vi "Initialize.vi"(8 "error in (no error)":errorcluster, 10 "Laser Configuration":T1, 11 "Coherent Laser in":refnum<class "Coherent Laser.lvclass">) -> (0 "error out":errorcluster, 3 "Coherent Laser out":refnum<class "Coherent Laser.lvclass">)   [LabVIEW 2023, in "Coherent Laser.lvlib" / "Coherent Laser.lvclass"]
uses:
  Coherent Laser.lvclass
  Resources/Type Defs/Laser Configuration.ctl
  Coherent Laser.lvclass/Coherent Laser.ctl
  Resources/GLOBAL/GLOBAL Debug.vi
  <vilib>/Utility/error.llb/Error Cluster From Error Code.vi
  <vilib>/ErrorRing/Error Ring.xnode
  <vilib>/Instr/_visa.llb/VISA Configure Serial Port (Instr).vi
  Coherent Laser.lvlib
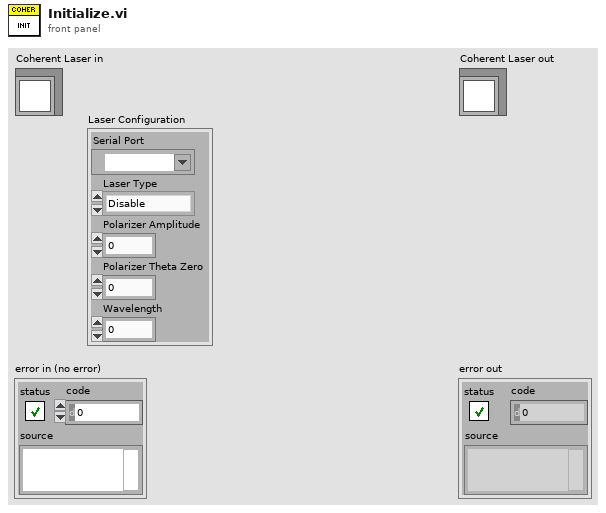
[diagram p1: front panel]
types:
  T1 = typedef "Laser Configuration.ctl" = cluster{"Serial Port":refnum<visa-resource-name>, "Laser Type":enum16{"Disable", "Laser Quantum", "Coherent OBIS", "PRM1-Z8", "Coherent HOPS"}, "Polarizer Amplitude":dbl, "Polarizer Theta Zero":dbl, "Wavelength":u16}
  T2 = enum16{"Disable", "Laser Quantum", "Coherent OBIS", "PRM1-Z8", "Coherent HOPS"}
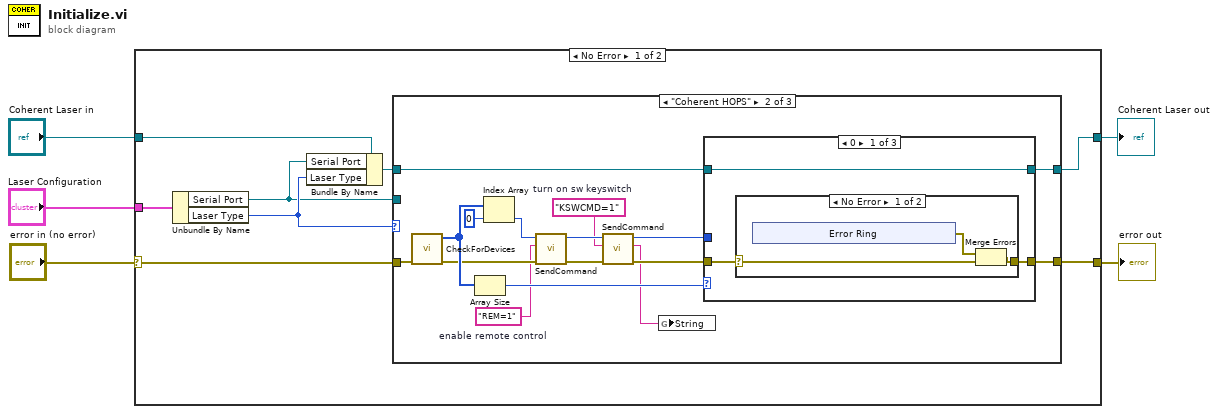
[diagram p0: block diagram]
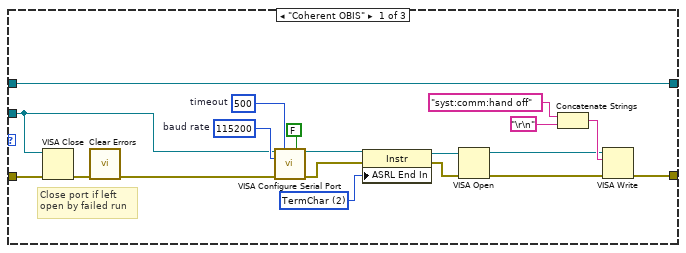
[diagram p2: hidden frame]
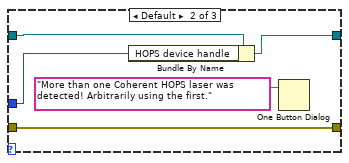
[diagram p4: hidden frame]
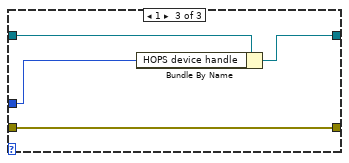
[diagram p5: hidden frame]
diagram:
  n1 = case shown="No Error" "error in (no error)" {
    selector: "error in (no error)" -> [w13 w72]
    tunnel: [w7 w72] -> w4
    tunnel: [w6 w71] -> w2
    tunnel: "Coherent Laser in" -> [w10 w71]
    tunnel: "Laser Configuration" -> [w12 _]
    frame No Error {
      n2 = Unbundle By Name(w12) -> ("Serial Port"=w8:refnum<visa-resource-name>, "Laser Type"=w9:T2)
      n3 = Bundle By Name(cluster=w10, "Serial Port"=w8, "Laser Type"=w9) -> (w11:refnum<class "Coherent Laser.lvclass">)
      n4 = case shown="\"Coherent HOPS\"" w9 {
        tunnel: w8 -> [w15 _ _]
        tunnel: w13 -> [w18 w48 w70]
        tunnel: [w27 w44 w70] -> w7
        tunnel: w11 -> [w14 w43 w69]
        tunnel: [w14 w42 w69] -> w6
        frame "Coherent OBIS" {
          w21 = u16 2 items=["None", "Last Bit", "TermChar"] ("Serial Settings:End Mode for Reads")
          w26 = u32 500  # timeout
          w28 = u32 115200  # baud rate
          # "Close port if left\nopen by failed run"
          n5 = VISA Close(VISA resource name=w15, error in (no error)=w18) -> (error out=w17:errorcluster)
          n6 = call <vilib>:"Clear Errors.vi"("error in (no error)"=w17) -> ("error out"=w16:errorcluster)  [unwired: 5 in, 1 out]
          n7 = call-poly "VISA Configure Serial Port"("VISA resource name"=w15, "timeout (10sec)"=w26, "Enable Termination\nChar (T)"=FALSE ("Enable Termination\nChar (T)"), "baud rate (9600)"=w28, "error in (no error)"=w16) -> ("VISA resource name out"=w25:refnum<visa-resource-name>, "error out"=w22:errorcluster)  [unwired: 9 in]
          n8 = property class="Instr"(reference=w25, error in=w22, "ASRL End In"=w21) -> (reference out=w24:refnum<visa-resource-name>, error out=w23:errorcluster)
          n9 = VISA Open(error in (no error)=w23, VISA resource name=w24) -> (VISA resource name=w19:refnum<visa-resource-name>, error out=w20:errorcluster)  [unwired: 3 in]
          n10 = Concatenate Strings("syst:comm:hand off" ("write to laser"), "\r\n") -> (w32:string)
          n11 = VISA Write(VISA resource name=w19, write buffer=w32, error in (no error)=w20) -> (error out=w27:errorcluster)  [unwired: 2 out]
        }
        frame "Coherent HOPS" {
          w33 = "KSWCMD=1"  # turn on sw keyswitch
          w39 = "REM=1"  # enable remote control
          n12 = call "CheckForDevices.vi"("error in"=w48) -> ("error out"=w41:errorcluster, "Device Handles"=w45:u64[])  [unwired: 6 in, 1 out]
          n13 = Array Size(array=w45) -> (size(s)=w46:i32)
          n14 = Index Array(array=w45, index=0 ("Index")) -> (element=w40:u64)
          n15 = call "SendCommand.vi"("error in"=w41, "Command"=w39, "Device Handle"=w40) -> ("error out"=w38:errorcluster, "Dup Handle"=w35:u64)  [unwired: 3 in, 2 out]
          n16 = call "SendCommand.vi"("error in"=w38, "Command"=w33, "Device Handle"=w35) -> ("error out"=w37:errorcluster, "String"=w34:string, "Dup Handle"=w36:u64)  [unwired: 3 in, 1 out]
          n17 = global write "GLOBAL Debug.vi" "String"(w34) -> ()
          n18 = case shown="0" w46 {
            tunnel: w36 -> [_ w60 w66]
            tunnel: w37 -> [w49 w63 w68]
            tunnel: [w51 w63 w68] -> w44
            tunnel: w43 -> [w50 w61 w67]
            tunnel: [w50 w62 w65] -> w42
            frame 0 {
              n19 = case shown="No Error" w49 {
                selector: w49 -> [w52 w59]
                tunnel: [w54 w59] -> w51
                frame No Error {
                  n20 = xnode "Error Ring"() -> ("error out"=w53:errorcluster)
                  n21 = Merge Errors(w53, w52) -> (w54:errorcluster)
                }
                frame Error {
                }
              }
            }
            frame Default {
              n22 = Bundle By Name(cluster=w61, "HOPS device handle"=w60) -> (w62:refnum<class "Coherent Laser.lvclass">)
              n23 = One Button Dialog(message="More than one Coherent HOPS laser was detected! Arbitrarily using the first.") -> ()  [unwired: 1 in, 1 out]
            }
            frame 1 {
              n24 = Bundle By Name(cluster=w67, "HOPS device handle"=w66) -> (w65:refnum<class "Coherent Laser.lvclass">)
            }
          }
        }
        frame Default {
        }
      }
    }
    frame Error {
    }
  }
  "error out" <- w4
  "Coherent Laser out" <- w2
